vi "scaler64.vi"(4 "divisor_Scaler":u32=1, 6 "PresetValues_Scaler":u32[](array[numeric])=[0, 0, 0, 0, 0, 0, 0, 0, 0, 0, 0, 0, 0, 0, 0, 0, 0, 0, 0, 0, 0, 0, 0, 0, 0, 0, 0, 0, 0, 0, 0, 0, 0, 0, 0, 0, 0, 0, 0, 0, 0, 0, 0, 0, 0, 0, 0, 0, 0, 0, 0, 0, 0, 0, 0, 0, 0, 0, 0, 0, 0, 0, 0, 0], 7 "AnalogInputs_Scaler":u32[](array[numeric])=[0, 0, 0, 0, 0, 0, 0, 0, 0, 0, 0, 0, 0, 0, 0, 0, 0, 0, 0, 0, 0, 0, 0, 0, 0, 0, 0, 0, 0, 0, 0, 0, 0, 0, 0, 0, 0, 0, 0, 0, 0, 0, 0, 0, 0, 0, 0, 0, 0, 0, 0, 0, 0, 0, 0, 0, 0, 0, 0, 0, 0, 0, 0], 8 "Pulse_Scaler":bool[](array[boolean])=[FALSE, FALSE, FALSE, FALSE, FALSE, FALSE, FALSE, FALSE, FALSE, FALSE, FALSE, FALSE, FALSE, FALSE, FALSE, FALSE, FALSE, FALSE, FALSE, FALSE, FALSE, FALSE, FALSE, FALSE, FALSE, FALSE, FALSE, FALSE, FALSE, FALSE, FALSE, FALSE, FALSE, FALSE, FALSE, FALSE, FALSE, FALSE, FALSE, FALSE, FALSE, FALSE, FALSE, FALSE, FALSE, FALSE, FALSE, FALSE, FALSE, FALSE, FALSE, FALSE, FALSE, FALSE, FALSE, FALSE, FALSE, FALSE, FALSE, FALSE, FALSE, FALSE, FALSE], 9 "OneShot_Scaler":bool, 10 "Gate_Scaler":bool[](array[boolean])=[FALSE, FALSE, FALSE, FALSE, FALSE, FALSE, FALSE, FALSE, FALSE, FALSE, FALSE, FALSE, FALSE, FALSE, FALSE, FALSE, FALSE, FALSE, FALSE, FALSE, FALSE, FALSE, FALSE, FALSE, FALSE, FALSE, FALSE, FALSE, FALSE, FALSE, FALSE, FALSE, FALSE, FALSE, FALSE, FALSE, FALSE, FALSE, FALSE, FALSE, FALSE, FALSE, FALSE, FALSE, FALSE, FALSE, FALSE, FALSE, FALSE, FALSE, FALSE, FALSE, FALSE, FALSE, FALSE, FALSE, FALSE, FALSE, FALSE, FALSE, FALSE, FALSE, FALSE, FALSE], 11 "Enable_Scaler":bool) -> (2 "Counter_Scaler":u32[](array[numeric]), 3 "Done_Scaler":bool)   [LabVIEW 2019, in "scaler.lvlib"]
uses:
  scaler.lvlib
  <vilib>/rvi/IPIntegrationNode/IPINode_Typedef/niFpgaIPINodeSupportedFamilies.ctl
  <vilib>/rvi/IPIntegrationNode/IPINode_Utilities/niFpgaIPINodeSimCore.vi
  <vilib>/rvi/IPIntegrationNode/IPINode_Xnode/niFpgaIPINode.xnode
  scaler_vhdl/src/Scaler64SimFiles/xsim.dir/scaler_64_lv_wrapper/xsimkE7343CD01BD446888FE8A1ECD56163F1.dll
panel:
  # "This is a 64 channel analog scaler. It follows to the word the definition of the scaler in the anl website\nhttps://epics.anl.gov/bcda/synApps/std/scalerRecord.html"
  # "This is the basic block for a scaler with 64 channels. It is used for the \ndigital, as well as the analog implementation of the scaler. The IP used\nwas implemented in VHDL and was verified using a simulation testbench."
  # "Input and output description\n - Gate_Scaler[64] : corresponds to 64 counters S1-S64\n - Pulse_Scaler[63] : corresponds to 63 counters S2-S64. The positive\n                                   edge of this signal is used to sum the AnalogInputs_Scaler\n                                   to the internal accumulation counters.\n - PresetValues_Scaler[64]: corresponds to 64 counters S1-S64\n - OneShot_Scaler: Oneshot / autocount is also implemented \n                                 in hardware. When necessary, can be used.\n                                 When not necessary (implmented in software)\n                                 this port can be fixed to 1.\n - AnalogInputs_Scaler[63] : The inputs to be summed when the\n                                                 corresponding Pulse_Scaler transits \n                                                 from 0 -> 1. (S2-S64)\n-  Divisor_Scaler: If not set to 1, the S1 counter will increment every\n                             \"Divisor\" ticks.\n - Counter_Scaler[64]: 64 counter readings.\n - Done_Scaler : Done signal as per Scaler specifications\n - Enable_Scaler: Set to one when CNT is set to 1."
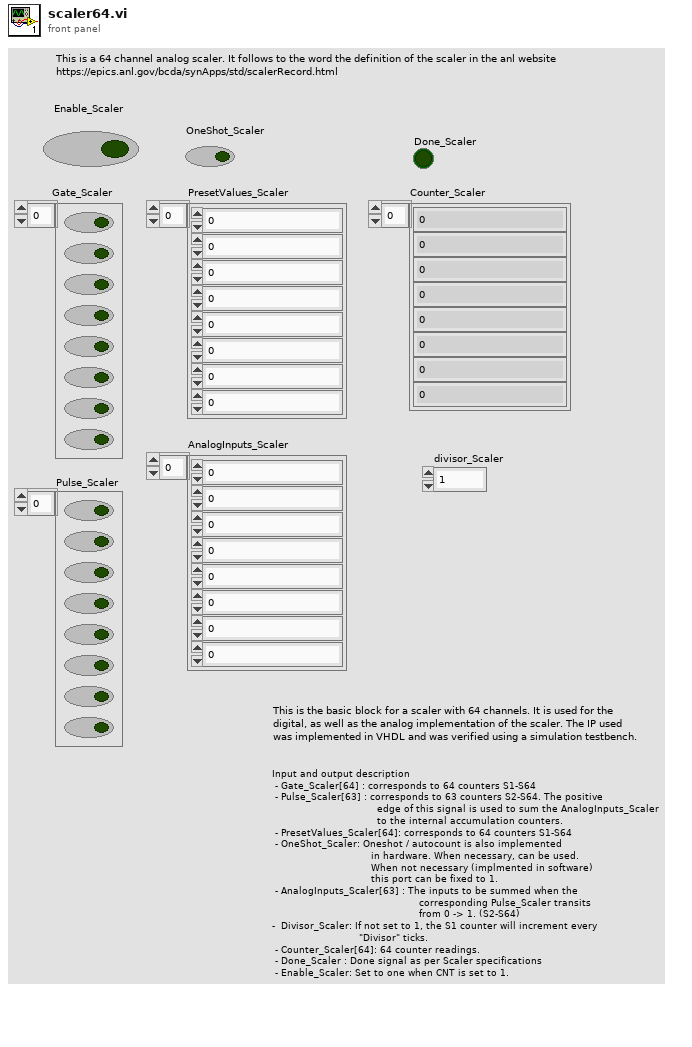
[diagram p1: front panel]
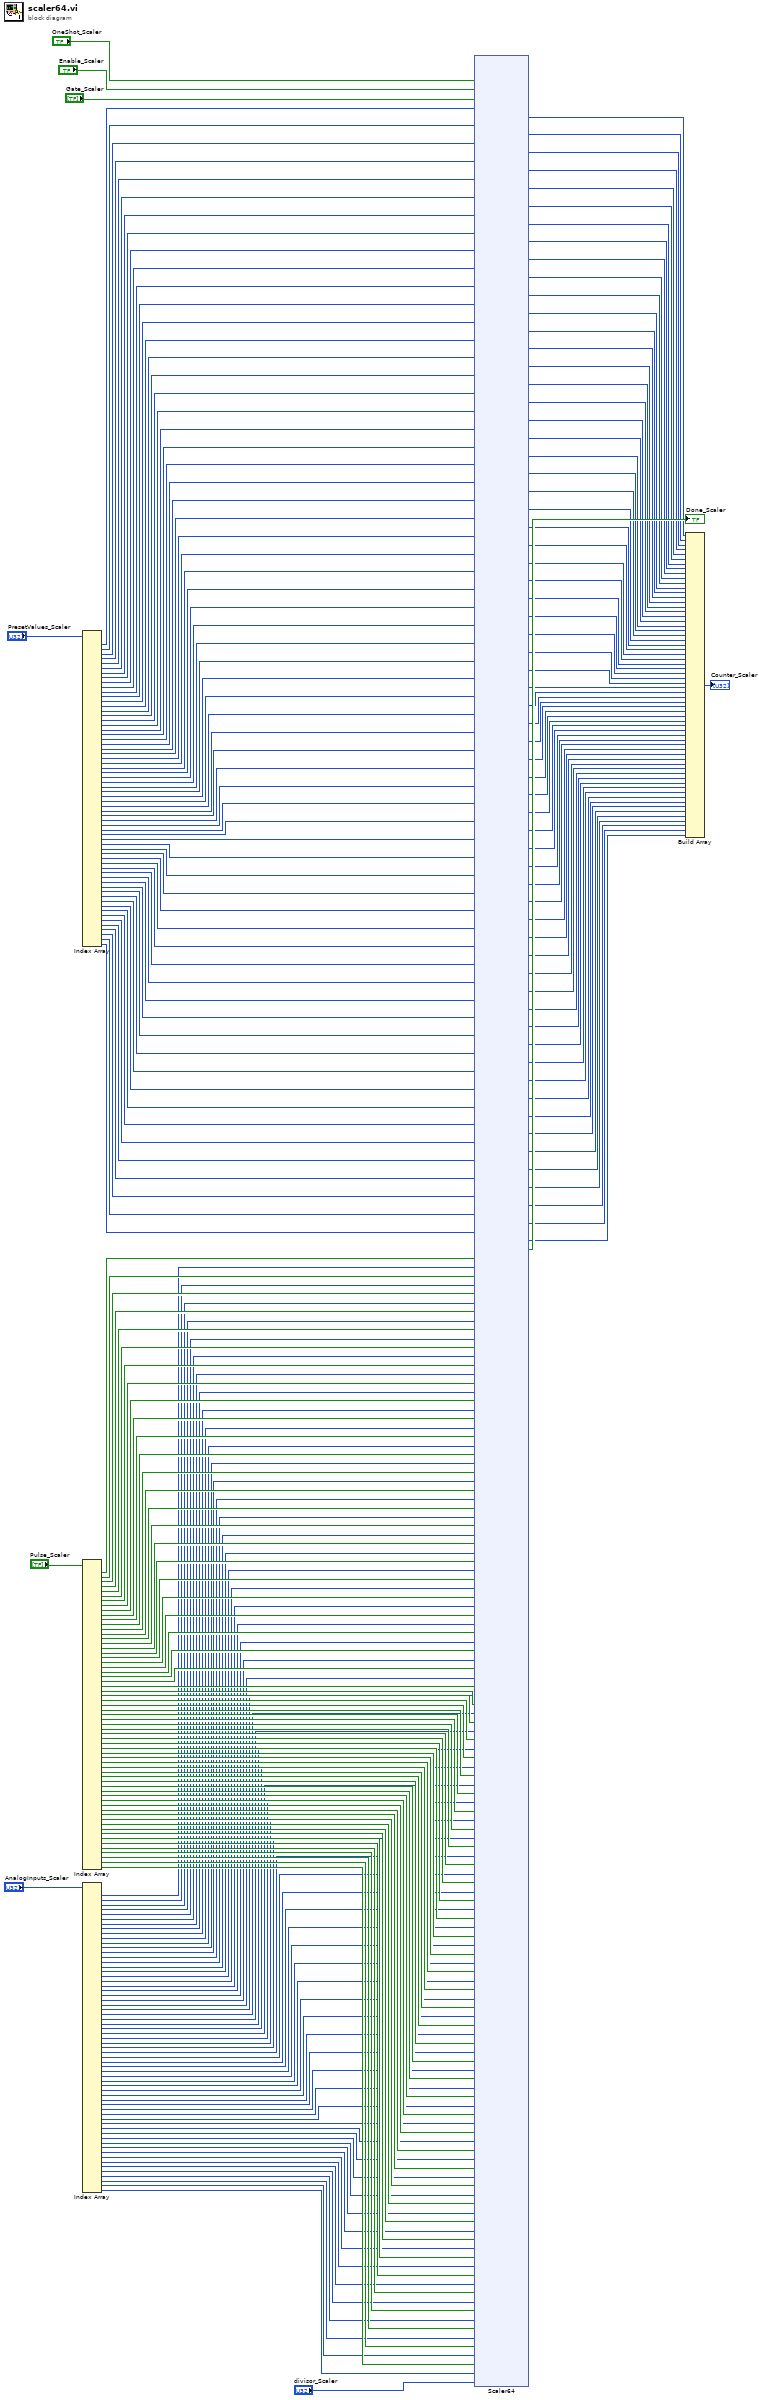
[diagram p0: block diagram]
diagram:
  n1 = Index Array(array="PresetValues_Scaler") -> (element #1=w259:u32, element #2=w258:u32, element #3=w257:u32, element #4=w256:u32, element #5=w255:u32, element #6=w254:u32, element #7=w253:u32, element #8=w252:u32, element #9=w251:u32, element #10=w250:u32, element #11=w249:u32, element #12=w248:u32, element #13=w247:u32, element #14=w246:u32, element #15=w245:u32, element #16=w244:u32, element #17=w243:u32, element #18=w242:u32, element #19=w241:u32, element #20=w240:u32, element #21=w239:u32, element #22=w238:u32, element #23=w237:u32, element #24=w236:u32, element #25=w235:u32, element #26=w234:u32, element #27=w233:u32, element #28=w232:u32, element #29=w231:u32, element #30=w230:u32, element #31=w229:u32, element #32=w228:u32, element #33=w227:u32, element #34=w226:u32, element #35=w225:u32, element #36=w224:u32, element #37=w223:u32, element #38=w222:u32, element #39=w221:u32, element #40=w220:u32, element #41=w219:u32, element #42=w218:u32, element #43=w217:u32, element #44=w216:u32, element #45=w215:u32, element #46=w214:u32, element #47=w213:u32, element #48=w212:u32, element #49=w211:u32, element #50=w210:u32, element #51=w209:u32, element #52=w208:u32, element #53=w207:u32, element #54=w206:u32, element #55=w205:u32, element #56=w204:u32, element #57=w203:u32, element #58=w202:u32, element #59=w201:u32, element #60=w200:u32, element #61=w199:u32, element #62=w198:u32, element #63=w197:u32, element #64=w196:u32)  [unwired: 64 in]
  n2 = Index Array(array="Pulse_Scaler") -> (element #1=w128:bool, element #2=w127:bool, element #3=w126:bool, element #4=w125:bool, element #5=w124:bool, element #6=w123:bool, element #7=w122:bool, element #8=w121:bool, element #9=w120:bool, element #10=w119:bool, element #11=w118:bool, element #12=w117:bool, element #13=w116:bool, element #14=w115:bool, element #15=w114:bool, element #16=w113:bool, element #17=w112:bool, element #18=w111:bool, element #19=w110:bool, element #20=w109:bool, element #21=w108:bool, element #22=w107:bool, element #23=w106:bool, element #24=w105:bool, element #25=w104:bool, element #26=w103:bool, element #27=w102:bool, element #28=w101:bool, element #29=w100:bool, element #30=w99:bool, element #31=w98:bool, element #32=w97:bool, element #33=w96:bool, element #34=w95:bool, element #35=w94:bool, element #36=w93:bool, element #37=w92:bool, element #38=w91:bool, element #39=w90:bool, element #40=w89:bool, element #41=w88:bool, element #42=w87:bool, element #43=w86:bool, element #44=w85:bool, element #45=w84:bool, element #46=w83:bool, element #47=w82:bool, element #48=w81:bool, element #49=w80:bool, element #50=w79:bool, element #51=w78:bool, element #52=w77:bool, element #53=w76:bool, element #54=w75:bool, element #55=w74:bool, element #56=w73:bool, element #57=w72:bool, element #58=w71:bool, element #59=w70:bool, element #60=w69:bool, element #61=w68:bool, element #62=w67:bool, element #63=w66:bool)  [unwired: 63 in]
  n3 = Index Array(array="AnalogInputs_Scaler") -> (element #1=w65:u32, element #2=w64:u32, element #3=w63:u32, element #4=w62:u32, element #5=w61:u32, element #6=w60:u32, element #7=w59:u32, element #8=w58:u32, element #9=w57:u32, element #10=w56:u32, element #11=w55:u32, element #12=w54:u32, element #13=w53:u32, element #14=w52:u32, element #15=w51:u32, element #16=w50:u32, element #17=w49:u32, element #18=w48:u32, element #19=w47:u32, element #20=w46:u32, element #21=w45:u32, element #22=w44:u32, element #23=w43:u32, element #24=w42:u32, element #25=w41:u32, element #26=w40:u32, element #27=w39:u32, element #28=w38:u32, element #29=w37:u32, element #30=w36:u32, element #31=w35:u32, element #32=w34:u32, element #33=w33:u32, element #34=w32:u32, element #35=w31:u32, element #36=w30:u32, element #37=w29:u32, element #38=w28:u32, element #39=w27:u32, element #40=w26:u32, element #41=w25:u32, element #42=w24:u32, element #43=w23:u32, element #44=w22:u32, element #45=w21:u32, element #46=w20:u32, element #47=w19:u32, element #48=w18:u32, element #49=w17:u32, element #50=w16:u32, element #51=w15:u32, element #52=w14:u32, element #53=w13:u32, element #54=w12:u32, element #55=w11:u32, element #56=w10:u32, element #57=w9:u32, element #58=w8:u32, element #59=w7:u32, element #60=w6:u32, element #61=w5:u32, element #62=w4:u32, element #63=w3:u32)  [unwired: 63 in]
  n4 = xnode ("Scaler64")("one_shot_i"="OneShot_Scaler", "scaler_enable_i"="Enable_Scaler", "gate_i"="Gate_Scaler", "preset_value_0_i"=w259, "preset_value_1_i"=w258, "preset_value_2_i"=w257, "preset_value_3_i"=w256, "preset_value_4_i"=w255, "preset_value_5_i"=w254, "preset_value_6_i"=w253, "preset_value_7_i"=w252, "preset_value_8_i"=w251, "preset_value_9_i"=w250, "preset_value_10_i"=w249, "preset_value_11_i"=w248, "preset_value_12_i"=w247, "preset_value_13_i"=w246, "preset_value_14_i"=w245, "preset_value_15_i"=w244, "preset_value_16_i"=w243, "preset_value_17_i"=w242, "preset_value_18_i"=w241, "preset_value_19_i"=w240, "preset_value_20_i"=w239, "preset_value_21_i"=w238, "preset_value_22_i"=w237, "preset_value_23_i"=w236, "preset_value_24_i"=w235, "preset_value_25_i"=w234, "preset_value_26_i"=w233, "preset_value_27_i"=w232, "preset_value_28_i"=w231, "preset_value_29_i"=w230, "preset_value_30_i"=w229, "preset_value_31_i"=w228, "preset_value_32_i"=w227, "preset_value_33_i"=w226, "preset_value_34_i"=w225, "preset_value_35_i"=w224, "preset_value_36_i"=w223, "preset_value_37_i"=w222, "preset_value_38_i"=w221, "preset_value_39_i"=w220, "preset_value_40_i"=w219, "preset_value_41_i"=w218, "preset_value_42_i"=w217, "preset_value_43_i"=w216, "preset_value_44_i"=w215, "preset_value_45_i"=w214, "preset_value_46_i"=w213, "preset_value_47_i"=w212, "preset_value_48_i"=w211, "preset_value_49_i"=w210, "preset_value_50_i"=w209, "preset_value_51_i"=w208, "preset_value_52_i"=w207, "preset_value_53_i"=w206, "preset_value_54_i"=w205, "preset_value_55_i"=w204, "preset_value_56_i"=w203, "preset_value_57_i"=w202, "preset_value_58_i"=w201, "preset_value_59_i"=w200, "preset_value_60_i"=w199, "preset_value_61_i"=w198, "preset_value_62_i"=w197, "preset_value_63_i"=w196, "pulse_1_i"=w128, "val_to_sum_1_i"=w65, "pulse_2_i"=w127, "val_to_sum_2_i"=w64, "pulse_3_i"=w126, "val_to_sum_3_i"=w63, "pulse_4_i"=w125, "val_to_sum_4_i"=w62, "pulse_5_i"=w124, "val_to_sum_5_i"=w61, "pulse_6_i"=w123, "val_to_sum_6_i"=w60, "pulse_7_i"=w122, "val_to_sum_7_i"=w59, "pulse_8_i"=w121, "val_to_sum_8_i"=w58, "pulse_9_i"=w120, "val_to_sum_9_i"=w57, "pulse_10_i"=w119, "val_to_sum_10_i"=w56, "pulse_11_i"=w118, "val_to_sum_11_i"=w55, "pulse_12_i"=w117, "val_to_sum_12_i"=w54, "pulse_13_i"=w116, "val_to_sum_13_i"=w53, "pulse_14_i"=w115, "val_to_sum_14_i"=w52, "pulse_15_i"=w114, "val_to_sum_15_i"=w51, "pulse_16_i"=w113, "val_to_sum_16_i"=w50, "pulse_17_i"=w112, "val_to_sum_17_i"=w49, "pulse_18_i"=w111, "val_to_sum_18_i"=w48, "pulse_19_i"=w110, "val_to_sum_19_i"=w47, "pulse_20_i"=w109, "val_to_sum_20_i"=w46, "pulse_21_i"=w108, "val_to_sum_21_i"=w45, "pulse_22_i"=w107, "val_to_sum_22_i"=w44, "pulse_23_i"=w106, "val_to_sum_23_i"=w43, "pulse_24_i"=w105, "val_to_sum_24_i"=w42, "pulse_25_i"=w104, "val_to_sum_25_i"=w41, "pulse_26_i"=w103, "val_to_sum_26_i"=w40, "pulse_27_i"=w102, "val_to_sum_27_i"=w39, "pulse_28_i"=w101, "val_to_sum_28_i"=w38, "pulse_29_i"=w100, "val_to_sum_29_i"=w37, "pulse_30_i"=w99, "val_to_sum_30_i"=w36, "pulse_31_i"=w98, "val_to_sum_31_i"=w35, "pulse_32_i"=w97, "val_to_sum_32_i"=w34, "pulse_33_i"=w96, "val_to_sum_33_i"=w33, "pulse_34_i"=w95, "val_to_sum_34_i"=w32, "pulse_35_i"=w94, "val_to_sum_35_i"=w31, "pulse_36_i"=w93, "val_to_sum_36_i"=w30, "pulse_37_i"=w92, "val_to_sum_37_i"=w29, "pulse_38_i"=w91, "val_to_sum_38_i"=w28, "pulse_39_i"=w90, "val_to_sum_39_i"=w27, "pulse_40_i"=w89, "val_to_sum_40_i"=w26, "pulse_41_i"=w88, "val_to_sum_41_i"=w25, "pulse_42_i"=w87, "val_to_sum_42_i"=w24, "pulse_43_i"=w86, "val_to_sum_43_i"=w23, "pulse_44_i"=w85, "val_to_sum_44_i"=w22, "pulse_45_i"=w84, "val_to_sum_45_i"=w21, "pulse_46_i"=w83, "val_to_sum_46_i"=w20, "pulse_47_i"=w82, "val_to_sum_47_i"=w19, "pulse_48_i"=w81, "val_to_sum_48_i"=w18, "pulse_49_i"=w80, "val_to_sum_49_i"=w17, "pulse_50_i"=w79, "val_to_sum_50_i"=w16, "pulse_51_i"=w78, "val_to_sum_51_i"=w15, "pulse_52_i"=w77, "val_to_sum_52_i"=w14, "pulse_53_i"=w76, "val_to_sum_53_i"=w13, "pulse_54_i"=w75, "val_to_sum_54_i"=w12, "pulse_55_i"=w74, "val_to_sum_55_i"=w11, "pulse_56_i"=w73, "val_to_sum_56_i"=w10, "pulse_57_i"=w72, "val_to_sum_57_i"=w9, "pulse_58_i"=w71, "val_to_sum_58_i"=w8, "pulse_59_i"=w70, "val_to_sum_59_i"=w7, "pulse_60_i"=w69, "val_to_sum_60_i"=w6, "pulse_61_i"=w68, "val_to_sum_61_i"=w5, "pulse_62_i"=w67, "val_to_sum_62_i"=w4, "pulse_63_i"=w66, "val_to_sum_63_i"=w3, "divisor_i"="divisor_Scaler") -> ("counter_0_o"=w194:u32, "counter_1_o"=w193:u32, "counter_2_o"=w192:u32, "counter_3_o"=w191:u32, "counter_4_o"=w190:u32, "counter_5_o"=w189:u32, "counter_6_o"=w188:u32, "counter_7_o"=w187:u32, "counter_8_o"=w186:u32, "counter_9_o"=w185:u32, "counter_10_o"=w184:u32, "counter_11_o"=w183:u32, "counter_12_o"=w182:u32, "counter_13_o"=w181:u32, "counter_14_o"=w180:u32, "counter_15_o"=w179:u32, "counter_16_o"=w178:u32, "counter_17_o"=w177:u32, "counter_18_o"=w176:u32, "counter_19_o"=w175:u32, "counter_20_o"=w174:u32, "counter_21_o"=w173:u32, "counter_22_o"=w172:u32, "counter_23_o"=w171:u32, "counter_24_o"=w170:u32, "counter_25_o"=w169:u32, "counter_26_o"=w168:u32, "counter_27_o"=w167:u32, "counter_28_o"=w166:u32, "counter_29_o"=w165:u32, "counter_30_o"=w164:u32, "counter_31_o"=w163:u32, "counter_32_o"=w162:u32, "counter_33_o"=w161:u32, "counter_34_o"=w160:u32, "counter_35_o"=w159:u32, "counter_36_o"=w158:u32, "counter_37_o"=w157:u32, "counter_38_o"=w156:u32, "counter_39_o"=w155:u32, "counter_40_o"=w154:u32, "counter_41_o"=w153:u32, "counter_42_o"=w152:u32, "counter_43_o"=w151:u32, "counter_44_o"=w150:u32, "counter_45_o"=w149:u32, "counter_46_o"=w148:u32, "counter_47_o"=w147:u32, "counter_48_o"=w146:u32, "counter_49_o"=w145:u32, "counter_50_o"=w144:u32, "counter_51_o"=w143:u32, "counter_52_o"=w142:u32, "counter_53_o"=w141:u32, "counter_54_o"=w140:u32, "counter_55_o"=w139:u32, "counter_56_o"=w138:u32, "counter_57_o"=w137:u32, "counter_58_o"=w136:u32, "counter_59_o"=w135:u32, "counter_60_o"=w134:u32, "counter_61_o"=w133:u32, "counter_62_o"=w132:u32, "counter_63_o"=w131:u32, "done_o"=→"Done_Scaler":bool)  [unwired: 2 in]
  n5 = Build Array(w194, w193, w192, w191, w190, w189, w188, w187, w186, w185, w184, w183, w182, w181, w180, w179, w178, w177, w176, w175, w174, w173, w172, w171, w170, w169, w168, w167, w166, w165, w164, w163, w162, w161, w160, w159, w158, w157, w156, w155, w154, w153, w152, w151, w150, w149, w148, w147, w146, w145, w144, w143, w142, w141, w140, w139, w138, w137, w136, w135, w134, w133, w132, w131) -> (→"Counter_Scaler":u32[])
